vi "Is Position on Right Half.vi"(10 "Position":cluster{"Left":i32, "Top":i32}, 11 "Monitor Bounds":T1) -> (3 "On Right?":bool)   [LabVIEW 2019, in "Peek Window.lvlib"]
uses:
  Peek Window.lvlib
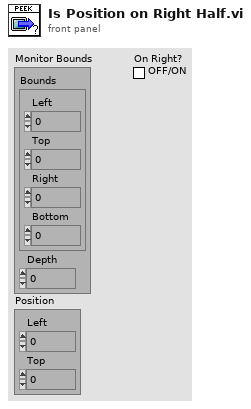
[diagram p1: front panel]
types:
  T1 = cluster{"Bounds":cluster{"Left":i16, "Top":i16, "Right":i16, "Bottom":i16}, "Depth":i16}
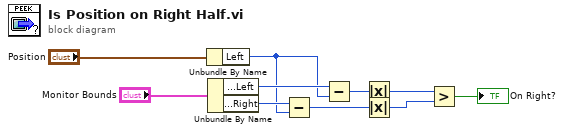
[diagram p0: block diagram]
diagram:
  n1 = Unbundle By Name("Position") -> ("Left"=w1:i32)
  n2 = Unbundle By Name("Monitor Bounds") -> ("Bounds.Left"=w4:i16, "Bounds.Right"=w5:i16)
  n3 = Subtract(x=w5, y=w1) -> (x-y=w7:i32)
  n4 = Subtract(x=w4, y=w1) -> (x-y=w6:i32)
  n5 = Absolute Value(x=w6) -> (abs(x)=w8:i32)
  n6 = Absolute Value(x=w7) -> (abs(x)=w9:i32)
  n7 = Greater?(x=w8, y=w9) -> (0:→"On Right?":bool)
